vi "PopulateTree(SubVI).vi"(0 "Tree Control reference":refnum<vi>, 1 "Array":T1[](array[typedef]), 2 "Display Neglected Status? (T)":bool=TRUE, 3 "Error In":errorcluster, 4 "Filter By AE Name":string) -> (10 "Error Out":errorcluster)   [LabVIEW 2017, in "DS_Lib.lvlib" / "SRReportParser.lvlib"]
uses:
  SRReportParser.lvlib
  TypeDefs/InWorkSR_Data.ctl
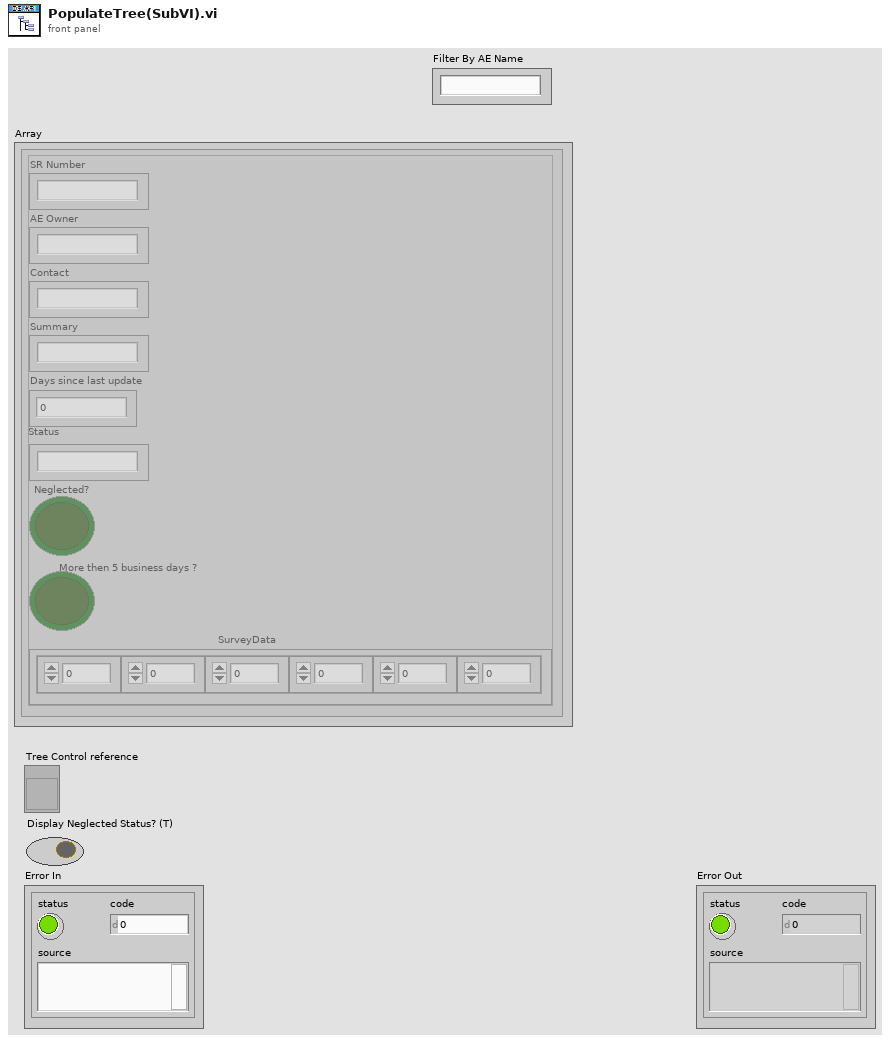
[diagram p1: front panel]
types:
  T1 = typedef "DS_Lib.lvlib/SRReportParser.lvlib/InWorkSR_Data.ctl" = cluster{"SR Number":string, "AE Owner":string, "Contact":string, "Summary":string, "Days since last update":dbl, "Status":string, "Neglected?":bool, "More then 5 business days ?":bool, "SurveyData":cluster{"Resolution Time":dbl, "Total Satisfaction":dbl, "Response Time":dbl, "Courtesy":dbl, "Problem Solved":dbl, "Level of effort":dbl}}
  T2 = cluster{"Left Cell String":string, "Child Text":string[], "Child Tag":string, "Item Indent":i32, "Child Only?":bool, "Glyph Index":i32}
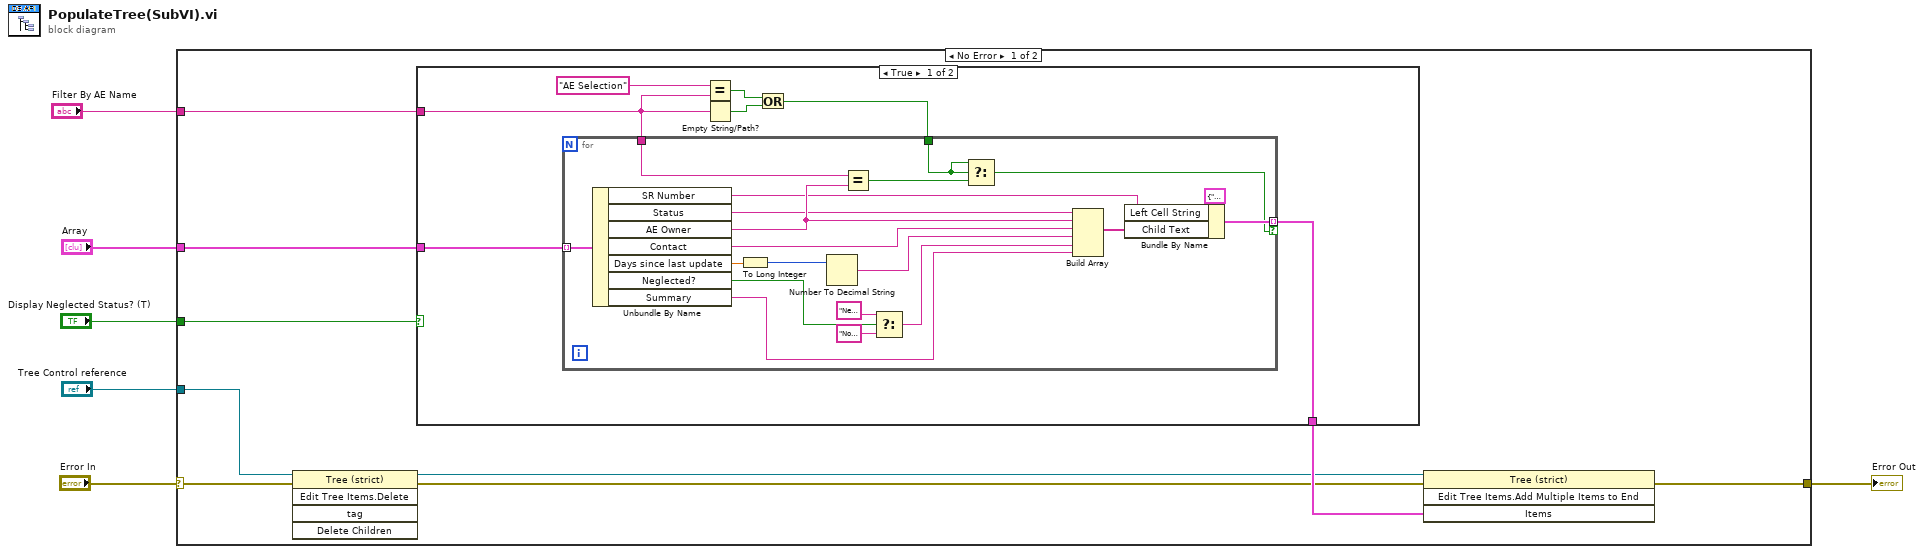
[diagram p0: block diagram]
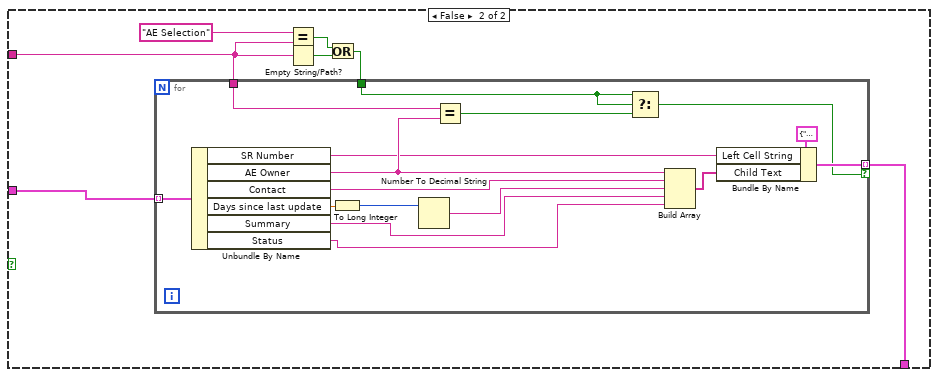
[diagram p2: hidden frame]
diagram:
  n1 = case shown="No Error" "Error In" {
    selector: "Error In" -> [w13 w66]
    tunnel: "Array" -> [w15 _]
    tunnel: "Filter By AE Name" -> [w14 _]
    tunnel: [w8 w66] -> w3
    tunnel: "Tree Control reference" -> [w12 _]
    tunnel: "Display Neglected Status? (T)" -> [w7 _]
    frame No Error {
      n2 = invoke on="Invoke Node" class="Tree (strict)" method="Edit Tree Items.Delete"(reference=w12, error in=w13) -> (reference out=w10:refnum<vi>, error out=w9:errorcluster)  [unwired: 3 in, 3 out]
      n3 = case shown="True" w7 {
        tunnel: w15 -> [w22 w49]
        tunnel: w14 -> [w18 w47]
        tunnel: [w21 w48] -> w11
        frame True {
          n4 = Equal?(x="AE Selection" ("String"), y=w18) -> (x = y?=w19:bool)
          n5 = Empty String/Path?(string/path=w18) -> (empty?=w16:bool)
          n6 = Or(x=w19, y=w16) -> (x .or. y?=w17:bool)
          n7 = for {
            tunnel: w22 -> [w42] mode=indexing
            tunnel: w18 -> [w31]
            tunnel: [w28] -> w21 mode=indexing if=w25
            tunnel: w17 -> [w27]
            n8 = Unbundle By Name(w42) -> ("SR Number"=w24:string, "Status"=w23:string, "AE Owner"=w32:string, "Contact"=w39:string, "Days since last update"=w41:dbl, "Neglected?"=w37:bool, "Summary"=w33:string)
            n9 = To Long Integer(number=w41) -> (32bit integer=w40:i32)
            n10 = Number To Decimal String(number=w40) -> (decimal integer string=w38:string)  [unwired: 1 in]
            n11 = Equal?(x=w31, y=w32) -> (x = y?=w26:bool)
            n12 = Select(t="Neglected" ("AE Owner"), s=w37, f="Not neglected" ("AE Owner")) -> (s? t:f=w34:string)
            n13 = Select(t=w27, s=w27, f=w26) -> (s? t:f=w25:bool)
            n14 = Build Array(w23, w32, w39, w38, w34, w33) -> (w29:string[])
            n15 = Bundle By Name(cluster=T2 {"Left Cell String"="", "Child Text"=[], "Child Tag"="", "Item Indent"=0, "Child Only?"=FALSE, "Glyph Index"=0} ("Item"), "Left Cell String"=w24, "Child Text"=w29) -> (w28:T2)
          }
        }
        frame False {
          n16 = Equal?(x="AE Selection" ("String"), y=w47) -> (x = y?=w44:bool)
          n17 = Empty String/Path?(string/path=w47) -> (empty?=w45:bool)
          n18 = Or(x=w44, y=w45) -> (x .or. y?=w43:bool)
          n19 = for {
            tunnel: w49 -> [w65] mode=indexing
            tunnel: w47 -> [w58]
            tunnel: [w54] -> w48 mode=indexing if=w51
            tunnel: w43 -> [w50]
            n20 = Unbundle By Name(w65) -> ("SR Number"=w56:string, "AE Owner"=w59:string, "Contact"=w62:string, "Days since last update"=w64:dbl, "Summary"=w60:string, "Status"=w53:string)
            n21 = To Long Integer(number=w64) -> (32bit integer=w63:i32)
            n22 = Number To Decimal String(number=w63) -> (decimal integer string=w61:string)  [unwired: 1 in]
            n23 = Equal?(x=w58, y=w59) -> (x = y?=w52:bool)
            n24 = Select(t=w50, s=w50, f=w52) -> (s? t:f=w51:bool)
            n25 = Build Array(w59, w62, w61, w60, w53) -> (w55:string[])
            n26 = Bundle By Name(cluster=T2 {"Left Cell String"="", "Child Text"=[], "Child Tag"="", "Item Indent"=0, "Child Only?"=FALSE, "Glyph Index"=0} ("Item"), "Left Cell String"=w56, "Child Text"=w55) -> (w54:T2)
          }
        }
      }
      n27 = invoke on="Invoke Node" class="Tree (strict)" method="Edit Tree Items.Add Multiple Items to End"(reference=w10, error in=w9, "Items"=w11) -> (error out=w8:errorcluster)  [unwired: 1 in, 3 out]
    }
    frame Error {
    }
  }
  "Error Out" <- w3
